vi "Go To Finishing Command.vi"(8 "error in (no error)":errorcluster, 11 "Command Processor in":refnum<class "Command Processor Actor.lvclass">) -> (0 "error out":errorcluster, 3 "State out":refnum<class "State Actor.lvclass">)   [LabVIEW 2014, in "Robot Actor Framework.lvlib" / "Command Processor Actor.lvlib" / "Command Processor Actor.lvclass"]
uses:
  Command Processor Actor.lvclass
  <vilib>/ni/Actors/State Actor/State Actor/State Actor.lvclass
  States/Finishing Command/Finishing Command.lvclass
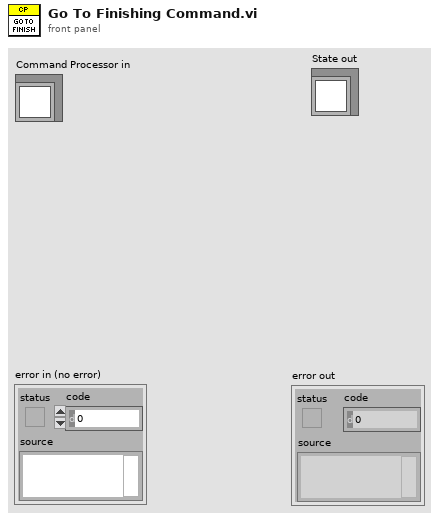
[diagram p1: front panel]
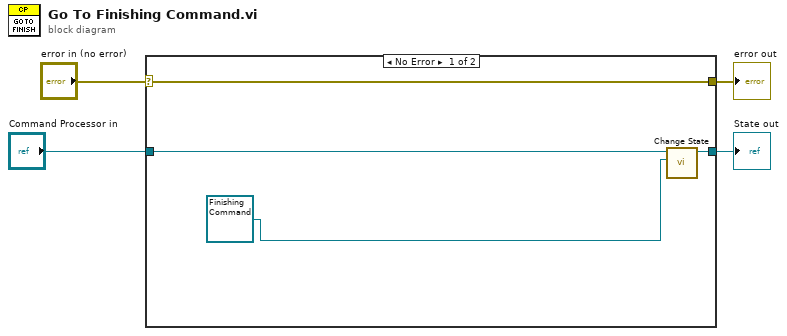
[diagram p0: block diagram]
diagram:
  n1 = case shown="No Error" "error in (no error)" {
    selector: "error in (no error)" -> [w8 w10]
    tunnel: [w8 w10] -> w3
    tunnel: [w7 w9] -> w1
    tunnel: "Command Processor in" -> [w6 w9]
    frame No Error {
      n2 = call <vilib>:"Change State.vi"("New State in"=refnum<class "Finishing Command.lvclass"> refnum ("Robot Actor Framework.lvlib:Command Processor Actor.lvlib:Finishing Command.lvclass"), "State in"=w6) -> ("State out"=w7:refnum<class "State Actor.lvclass">)  [unwired: 8 in, 1 out]
    }
    frame Error {
    }
  }
  "error out" <- w3
  "State out" <- w1
